vi "to INT8.vi"(8 "error in":errorcluster, 11 "bytes":u8[](array[numeric]) format="%b") -> (0 "error out":errorcluster, 2 "INT8":i8, 3 "remaining bytes":u8[](array[numeric]))   [LabVIEW 2020, in "MessagePack.lvlib" / "MessagePack.lvclass"]
uses:
  MessagePack.lvclass
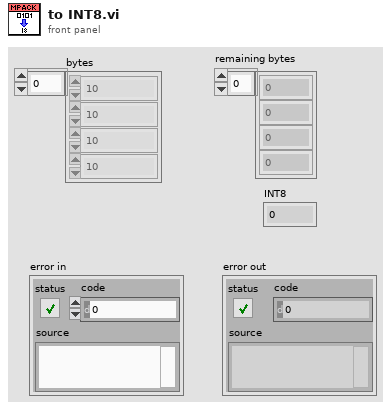
[diagram p1: front panel]
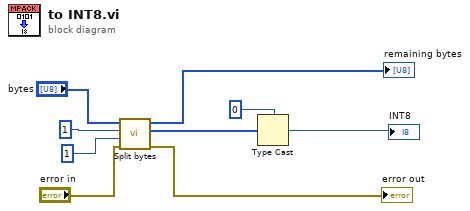
[diagram p0: block diagram]
diagram:
  n1 = call "Split bytes.vi"("error in"="error in", "End index"=1, "Start index"=1 ("minimum number"), "bytes in"="bytes") -> ("error out"=→"error out":errorcluster, "selected bytes"=w2:u8[], "remaining bytes"=→"remaining bytes":u8[])  [unwired: 4 in, 1 out]
  n2 = Type Cast(type=i8 0 ("INT8"), x=w2) -> (*(type *) &x=→"INT8":i8)
